vi "Lift E Stop.vi"   [LabVIEW 2014]
uses:
  Begin/Global Variables.vi
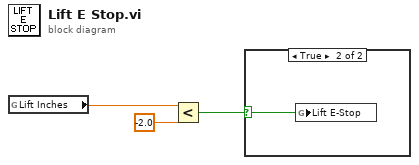
[diagram p0: block diagram]
diagram:
  n1 = global read "Global Variables.vi" "Lift Inches"() -> (w1:dbl)
  n2 = Less?(x=w1, y=-2.0) -> (x < y?=w2:bool)
  n3 = case shown="True" w2 {
    selector: w2 -> [_ w4]
    frame False {
    }
    frame True {
      n4 = global write "Global Variables.vi" "Lift E-Stop"(w4) -> ()
    }
  }
